vi "CopyFont.vi"(8 "error in (no error)":errorcluster, 11 "Application in":refnum<class "Game.lvclass">) -> (0 "error out":errorcluster, 3 "Application out":refnum<class "Game.lvclass">)   [LabVIEW 2021, in "Game.lvclass"]
uses:
  Game.lvclass
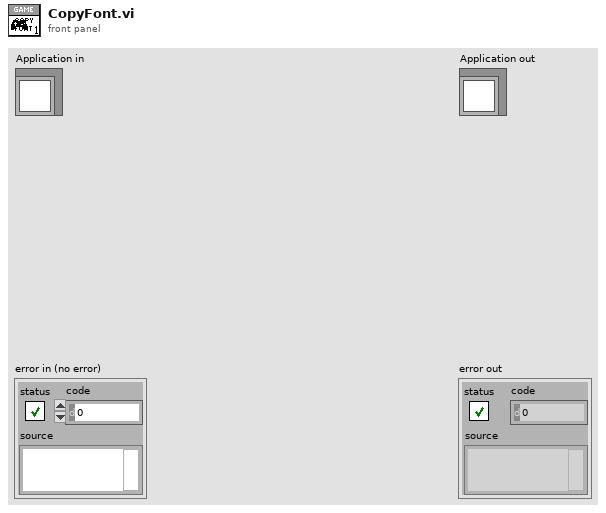
[diagram p1: front panel]
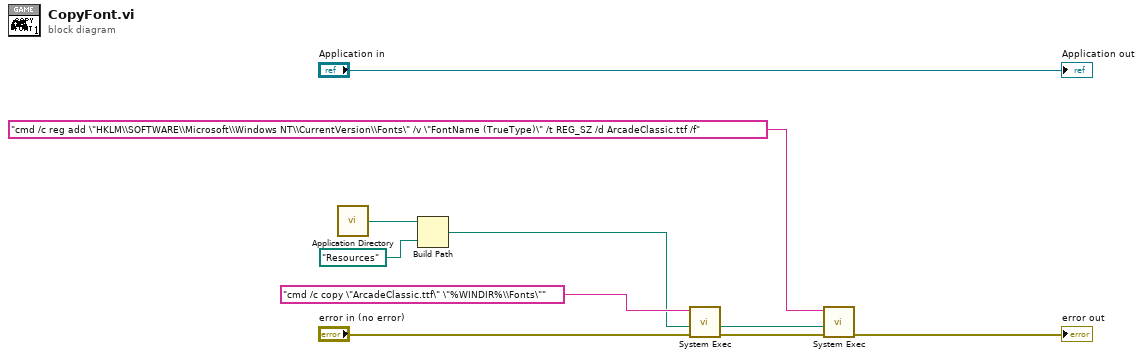
[diagram p0: block diagram]
diagram:
  n1 = call <vilib>:"Application Directory.vi"() -> ("Application Directory"=w7:path)
  n2 = Build Path(base path=w7, name or relative path=path "Resources") -> (appended path=w4:path)
  n3 = call <vilib>:"System Exec.vi"("error in (no error)"="error in (no error)", "working directory"=w4, "command line"="cmd /c copy \"ArcadeClassic.ttf\" \"%WINDIR%\\Fonts\"") -> ("error out"=w2:errorcluster)  [unwired: 5 in, 3 out]
  n4 = call <vilib>:"System Exec.vi"("error in (no error)"=w2, "working directory"=w4, "command line"="cmd /c reg add \"HKLM\\SOFTWARE\\Microsoft\\Windows NT\\CurrentVersion\\Fonts\" /v \"FontName (TrueType)\" /t REG_SZ /d ArcadeClassic.ttf /f") -> ("error out"=→"error out":errorcluster)  [unwired: 5 in, 3 out]
  "Application out" <- "Application in"
